vi "Joystick Read.vi"(8 "error in":errorcluster, 11 "Joystick In":T2) -> (0 "error out":errorcluster, 1 "POVs":i16[](array[numeric]), 2 "Buttons":T1, 3 "Axes":dbl[](array[numeric]))   [LabVIEW 2015]
uses:
  Joystick Info.ctl
  <vilib>/Rock Robotics/WPI/Joystick/WPI_JoystickDevRef.ctl
  <vilib>/Rock Robotics/WPI/Joystick/WPI_JoystickDeviceEnum.ctl
  Motors/Control 3.ctl
panel:
  out "Joystick Out":T2
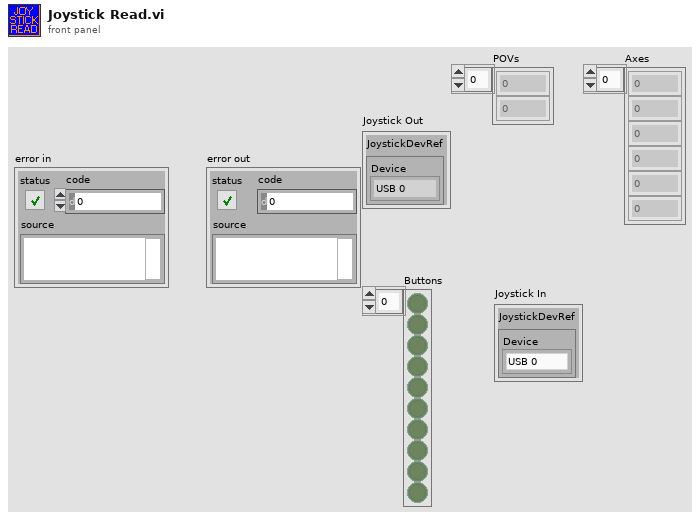
[diagram p1: front panel]
types:
  T1 = typedef "Control 3.ctl" = bool[]
  T2 = typedef "Joystick Info.ctl" = cluster{"JoystickDevRef":T3}
  T3 = typedef "WPI_JoystickDevRef.ctl" = cluster{"Device":T4}
  T4 = typedef "WPI_JoystickDeviceEnum.ctl" = enum16{"USB 0", "USB 1", "USB 2", "USB 3", "USB 4", "USB 5"}
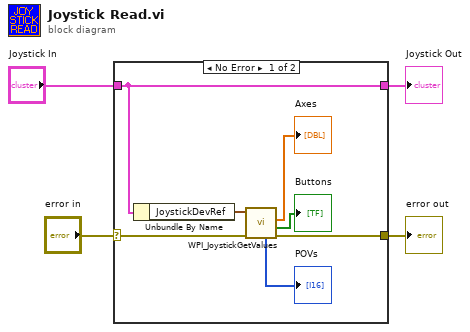
[diagram p0: block diagram]
diagram:
  n1 = case shown="No Error" "error in" {
    selector: "error in" -> [w7 w13]
    tunnel: [w6 w13] -> w3
    tunnel: "Joystick In" -> [w10 w12]
    tunnel: [w10 w12] -> w1
    frame No Error {
      n2 = Unbundle By Name(w10) -> ("JoystickDevRef"=w11:T3)
      n3 = call <vilib>:"WPI_JoystickGetValues.vi"("error in (no error)"=w7, "JoystickDevRef"=w11) -> ("error out"=w6:errorcluster, "Buttons"=→"Buttons":bool[], "Axes"=→"Axes":dbl[], "POVs"=→"POVs":i16[])  [unwired: 5 in, 1 out]
    }
    frame Error {
    }
  }
  "error out" <- w3
  "Joystick Out" <- w1
